vi "TH2829-20查询结果.vi"(7 "显示格式":enum16{"浮点计数法", "科学计数法"}(ring), 8 "error in":errorcluster caption="错误输入（无错误）", 9 "数量级":T1) -> (0 "error out":errorcluster caption="错误输出", 2 "judge":u8[][][](array[numeric]), 3 "result":string[][][](array[string]))   [LabVIEW 2018]
panel:
  out "read buffer":string
  out "Serial Settings:Number of Bytes at Serial Port":u32
  in  "仪器通讯端口":refnum<visa-resource-name>
  out "LED IrCompare Result":u8[][](array[numeric])
  out "LED IrResult":sgl[][](array[numeric]) format="%#_6f"
  out "总判断":u8
  out "Bls Result":sgl[][](array[numeric]) format="%#_6f"
  out "LED VfCompare Result":u8[][](array[numeric])
  out "LED VfResult":sgl[][](array[numeric]) format="%#_6f"
  out "TURN判断组合":u8[][](array[numeric])
  out "TURN数据组合":string[][](array[string])
  out "PS Compare Result":u8[][](array[numeric])
  out "Polarity Result1":string[][](array[string])
  out "Rs Compare Result":u8[][](array[numeric])
  out "Z Compare Result":u8[][](array[numeric])
  out "Balance Compare Result":u8[][](array[numeric])
  out "LxQ Compare Result":u8[][](array[numeric])
  out "DCR Compare Result":u8[][](array[numeric])
  out "C Compare Result":u8[][](array[numeric])
  out "Lk Compare Result":u8[][](array[numeric])
  out "Lx Compare Result":u8[][](array[numeric])
  out "Turns Compare Result":u8[][](array[numeric])
  out "Polarity Result":u8[][](array[numeric])
  out "Zx Result":sgl[][](array[numeric]) format="%#_6f"
  out "ACR Result":sgl[][](array[numeric]) format="%#_6f"
  out "LxQ Result":sgl[][](array[numeric]) format="%#_6f"
  out "DCR Result":sgl[][](array[numeric]) format="%#_6f"
  out "Cx Result":sgl[][](array[numeric]) format="%#_6f"
  out "Lk Result":sgl[][](array[numeric]) format="%#_6f"
  out "Lx Result":sgl[][](array[numeric]) format="%#_6f"
  out "Turns Result":sgl[][](array[numeric]) format="%#_6f"
  out "Primary Sets":string
  out "head":string
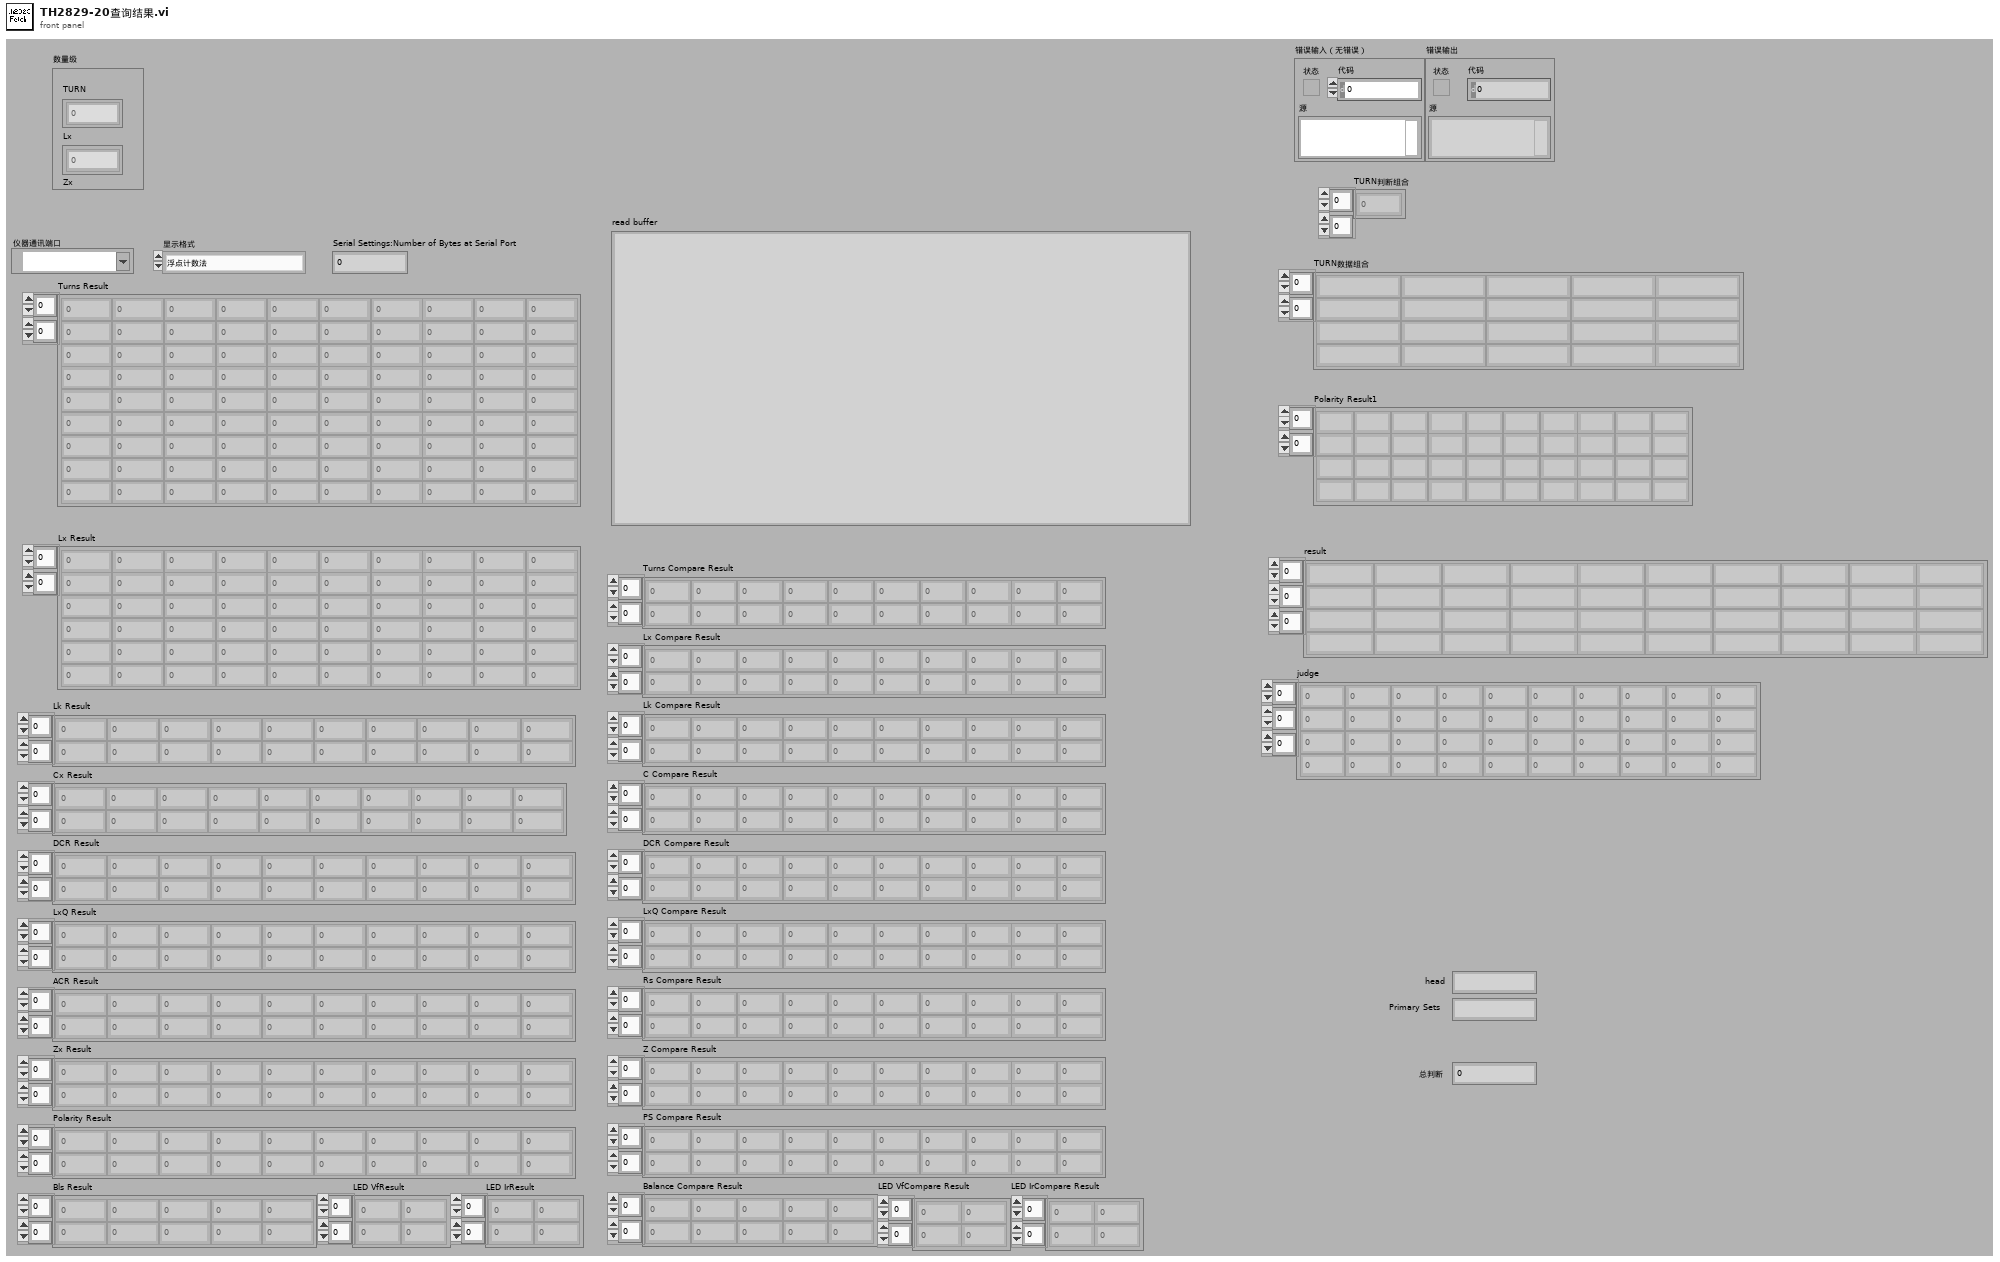
[diagram p1: front panel]
types:
  T1 = cluster{"TURN":sgl[][], "Lx":sgl[][], "Zx":sgl[][], "LK":sgl[][], "Cx":sgl[][], "ACR":sgl[][], "DCR":sgl[][], "LED+":sgl[][], "LED-":sgl[][]}
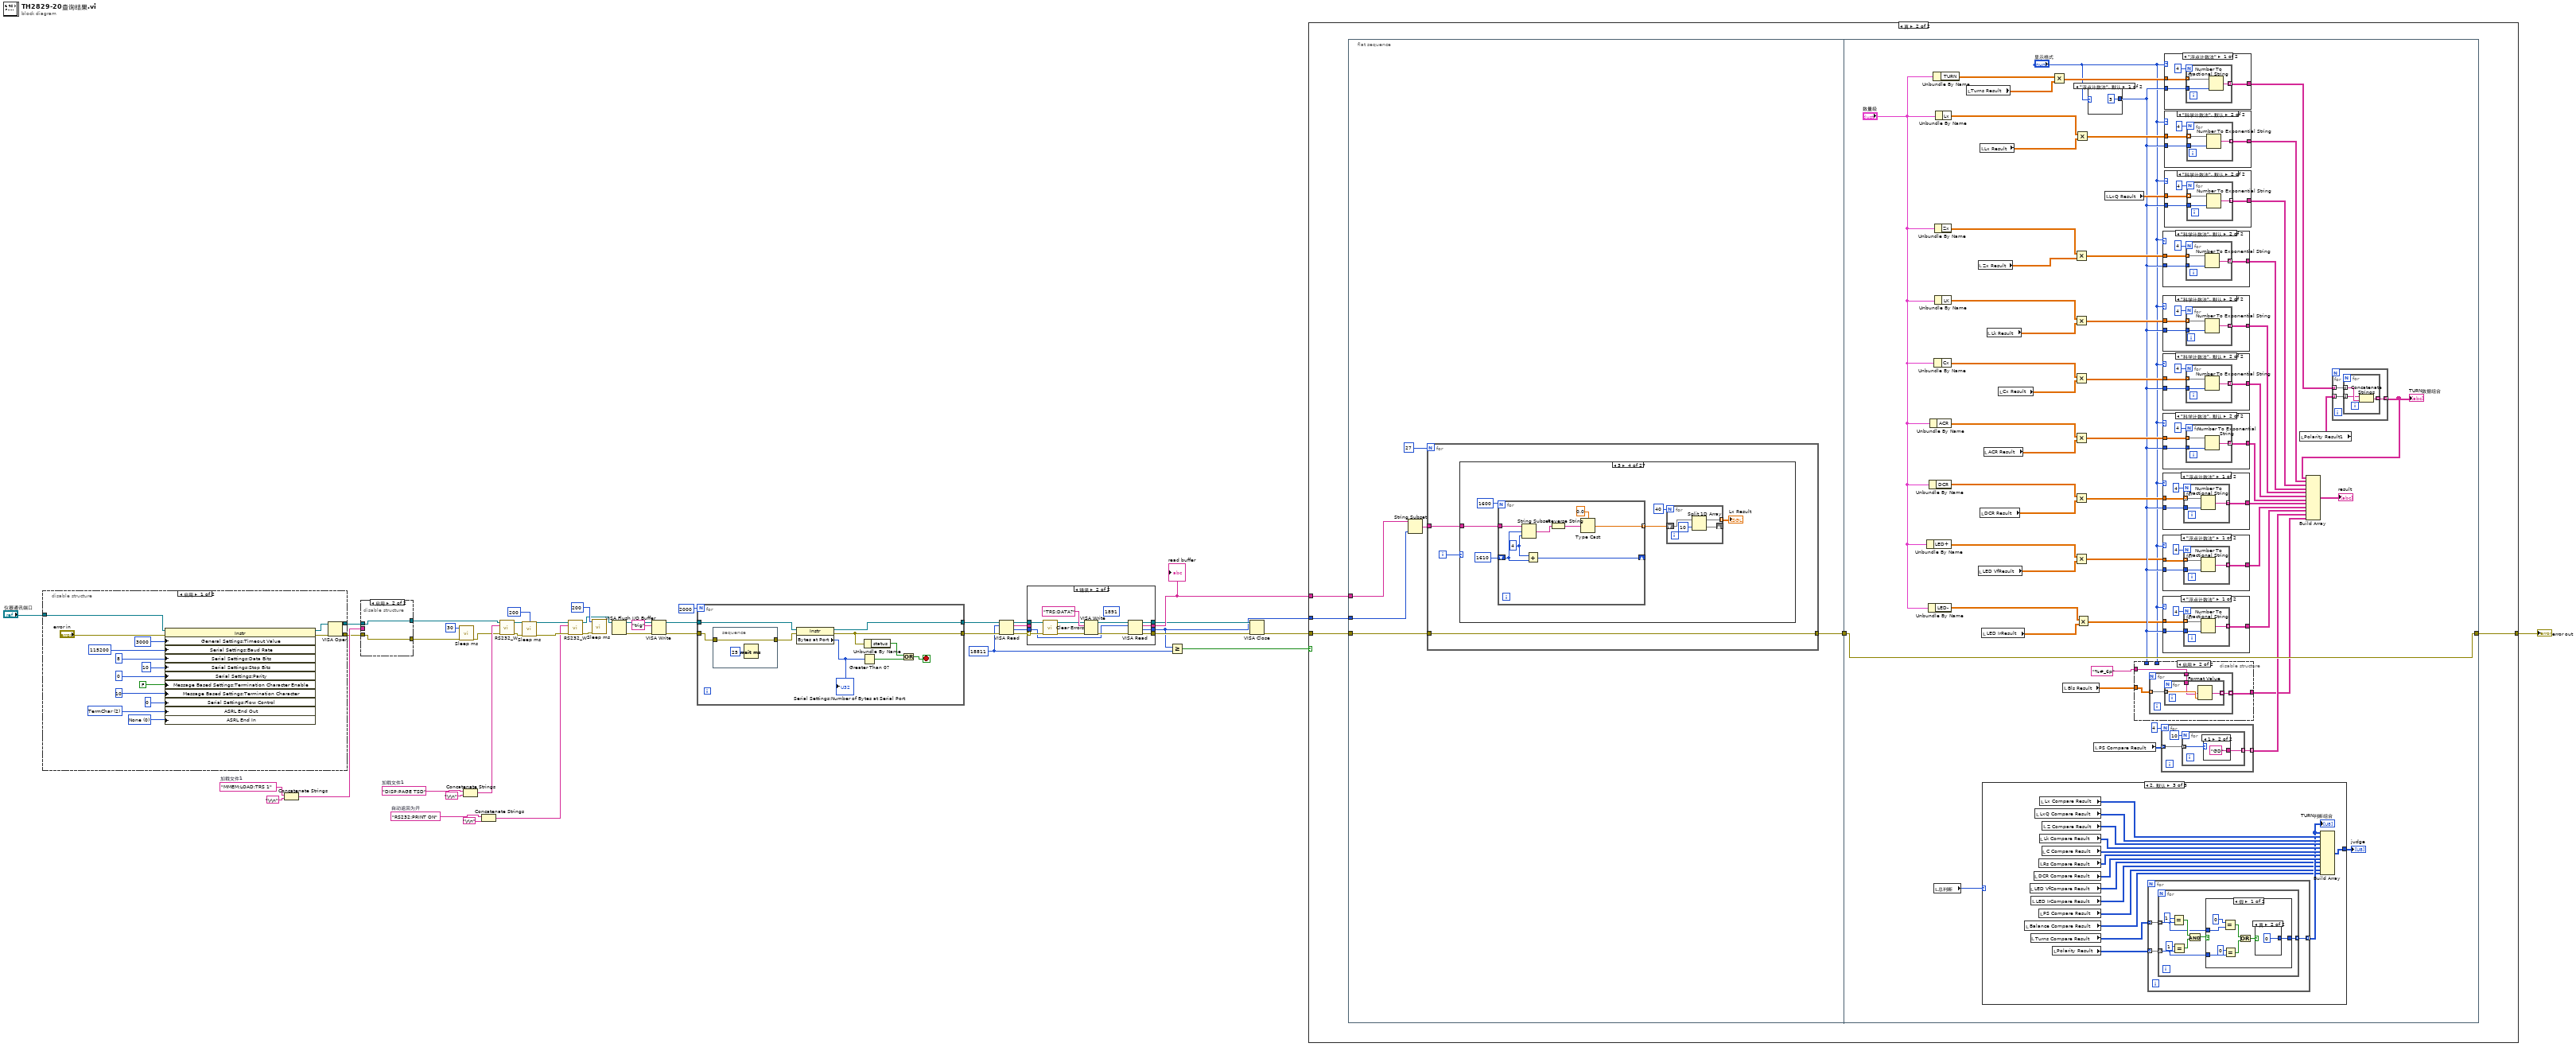
[diagram p0: block diagram]
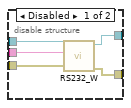
[diagram p2: hidden frame]
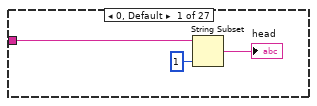
[diagram p6: hidden frame]
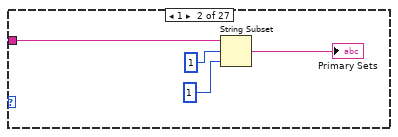
[diagram p7: hidden frame]
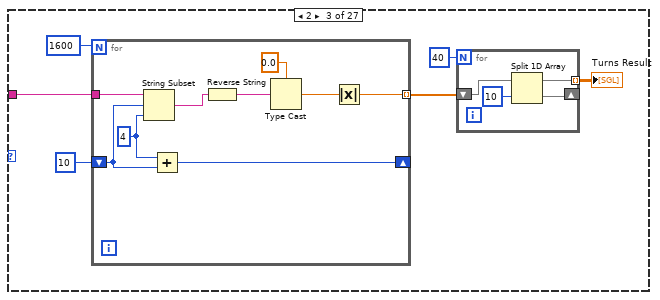
[diagram p8: hidden frame]
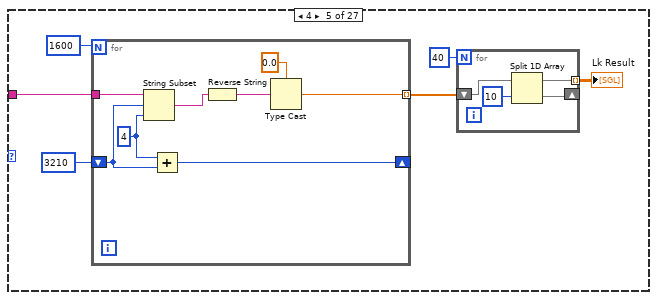
[diagram p9: hidden frame]
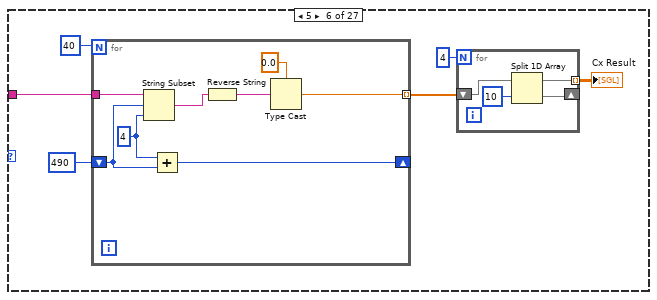
[diagram p10: hidden frame]
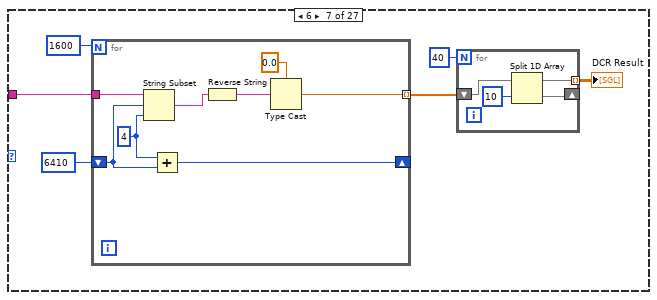
[diagram p11: hidden frame]
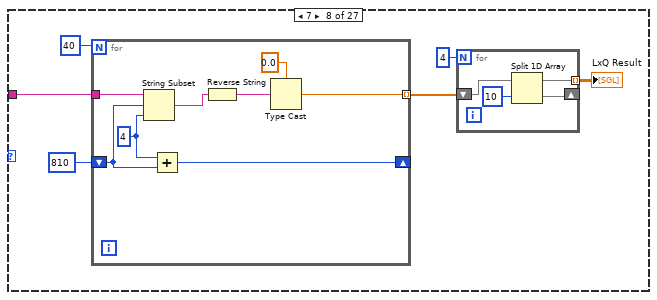
[diagram p12: hidden frame]
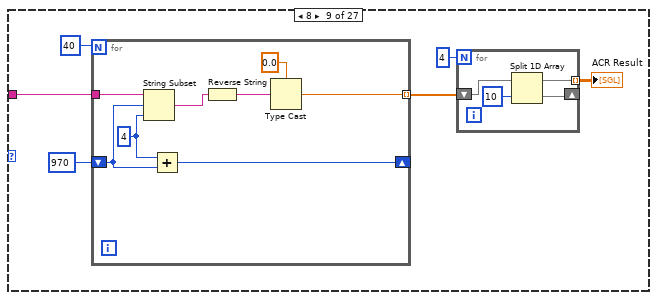
[diagram p13: hidden frame]
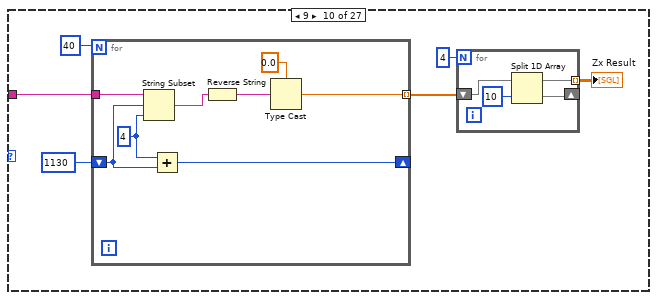
[diagram p14: hidden frame]
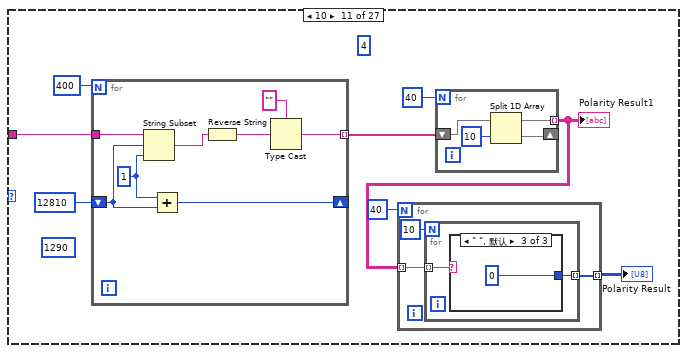
[diagram p15: hidden frame]
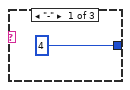
[diagram p16: hidden frame]
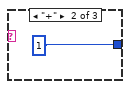
[diagram p17: hidden frame]
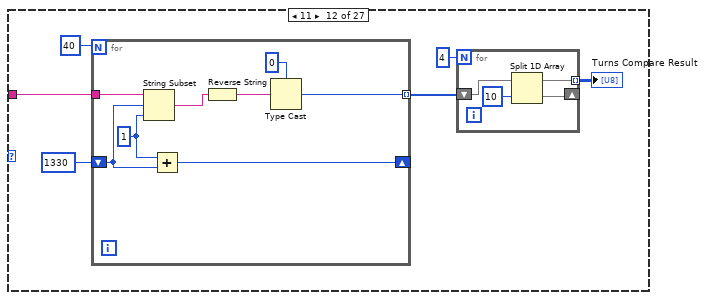
[diagram p18: hidden frame]
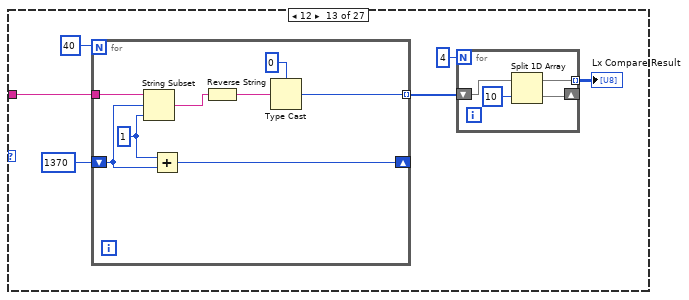
[diagram p19: hidden frame]
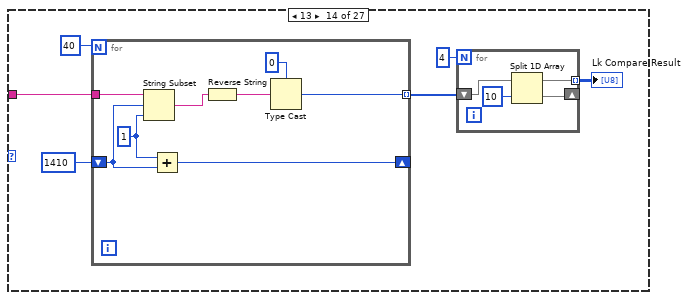
[diagram p20: hidden frame]
diagram:
  w8 = "MMEM:LOAD:TRS 1"  # 加载文件1
  w10 = "RS232:PRINT ON"  # 自动返回为开
  w11 = "DISP:PAGE TSD"  # 加载文件1
  w29 = u32 18811 ("字节总数")
  n1 = disable-structure shown="启用" {
    disable-tunnel: [w59 w60] -> w6
    disable-tunnel: [w58 _] -> w5
    disable-tunnel: "仪器通讯端口" -> [w55 w60]
    frame Enabled {
      w48 = u16 0 items=["None", "Last Bit", "TermChar"] ("Serial Settings:End Mode for Reads")
      w50 = u16 2 items=["None", "Last Bit", "TermChar", "Break"] ("Serial Settings:End Mode for Writes")
      n2 = property class="Instr"(reference=w55, error in="error in", "General Settings:Timeout Value"=u32 3000, "Serial Settings:Baud Rate"=u32 115200, "Serial Settings:Data Bits"=u16 8, "Serial Settings:Stop Bits"=u16 10, "Serial Settings:Parity"=u16 0, "Message Based Settings:Termination Character Enable"=FALSE ("TermChar En"), "Message Based Settings:Termination Character"=u8 10, "Serial Settings:Flow Control"=u16 0, "ASRL End Out"=w50, "ASRL End In"=w48) -> (reference out=w56:refnum<visa-resource-name>, error out=w57:errorcluster)
      n3 = VISA Open ("VISA打开")(error in (no error)=w57, VISA resource name=w56) -> (VISA resource name=w59:refnum<visa-resource-name>, error out=w58:errorcluster)  [unwired: 3 in]
    }
    frame Disabled {
    }
  }
  n4 = Concatenate Strings(w8, "\r\n") -> (w7:string)
  n5 = disable-structure shown="启用" {
    disable-tunnel: w7 -> [w65 _]
    disable-tunnel: w6 -> [w64 w67]
    disable-tunnel: w5 -> [w63 w66]
    disable-tunnel: [w62 w66] -> w4
    disable-tunnel: [w61 w67] -> w2
    frame Disabled {
      n6 = call "RS232_W.vi"("error in (no error)"=w63, "CMD"=w65, "VISA资源名称"=w64) -> ("error out"=w62:errorcluster, "VISA资源名称输出"=w61:refnum<visa-resource-name>)  [unwired: 6 in, 1 out]
    }
    frame Enabled {
    }
  }
  n7 = call "Sleep ms.vi"("error in (no error)"=w4, "等待时间（毫秒）"=u32 30) -> ("error out"=w1:errorcluster)  [unwired: 9 in]
  n8 = Concatenate Strings(w11, "\r\n") -> (w16:string)
  n9 = Concatenate Strings(w10, "\r\n") -> (w14:string)
  n10 = call "RS232_W.vi"("error in (no error)"=w1, "CMD"=w16, "VISA资源名称"=w2) -> ("error out"=w20:errorcluster, "VISA资源名称输出"=w17:refnum<visa-resource-name>)  [unwired: 6 in, 1 out]
  n11 = call "Sleep ms.vi"("error in (no error)"=w20, "等待时间（毫秒）"=u32 200) -> ("error out"=w21:errorcluster)  [unwired: 9 in]
  n12 = call "RS232_W.vi"("error in (no error)"=w21, "CMD"=w14, "VISA资源名称"=w17) -> ("error out"=w18:errorcluster, "VISA资源名称输出"=w13:refnum<visa-resource-name>)  [unwired: 6 in, 1 out]
  n13 = call "Sleep ms.vi"("error in (no error)"=w18, "等待时间（毫秒）"=u32 200) -> ()  [unwired: 9 in, 1 out]
  n14 = VISA Flush I/O Buffer(VISA resource name=w13) -> (VISA resource name out=w36:refnum<visa-resource-name>, error out=w37:errorcluster)  [unwired: 2 in]
  n15 = VISA Write(VISA resource name=w36, write buffer="trig", error in (no error)=w37) -> (VISA resource name out=w31:refnum<visa-resource-name>, error out=w32:errorcluster)  [unwired: 1 out]
  n16 = for {
    N: 2000 -> [_]
    tunnel: w31 -> [w76]
    tunnel: w32 -> [w68]
    tunnel: [w75] -> w34
    tunnel: [w72] -> w33
    stop <- w70 stop-if-true
    n17 = stacked-sequence {
      tunnel: [w78] -> w69
      tunnel: w68 -> [w78]
      frame #0 {
        n18 = Wait (ms)(milliseconds to wait=u32 25 ("等待时间（毫秒）")) -> ()  [unwired: 1 out]
      }
    }
    n19 = property class="Instr"(reference=w76, error in=w69) -> (reference out=w75:refnum<visa-resource-name>, error out=w72:errorcluster, "Bytes at Port"=w74:u32)
    "Serial Settings:Number of Bytes at Serial Port" <- w74
    n20 = Greater Than 0?(x=w74) -> (x > 0?=w73:bool)
    n21 = Unbundle By Name(w72) -> ("status"=w71:bool)
    n22 = Or(x=w71, y=w73) -> (x .or. y?=w70:bool)
  }
  n23 = VISA Read(VISA resource name=w34, byte count=w29, error in (no error)=w33) -> (VISA resource name out=w27:refnum<visa-resource-name>, read buffer=w25:string, return count=w26:u32, error out=w28:errorcluster)
  n24 = case shown="错误" w28 {
    selector: w28 -> [w82 w89]
    tunnel: w27 -> [w81 w88]
    tunnel: [w81 w87] -> w38
    tunnel: [w82 w86] -> w39
    tunnel: [w79 w85] -> w40
    tunnel: [w80 w84] -> w24
    tunnel: w26 -> [w80 w83]
    tunnel: w25 -> [w79 _]
    frame No Error {
    }
    frame Error {
      (unwired) u32 1891 ("字节总数")
      n25 = call <vilib>:"Clear Errors.vi"("error in (no error)"=w89) -> ("error out"=w90:errorcluster)  [unwired: 5 in, 1 out]
      n26 = VISA Write(VISA resource name=w88, write buffer="TRS:DATA?", error in (no error)=w90) -> (VISA resource name out=w92:refnum<visa-resource-name>, error out=w93:errorcluster)  [unwired: 1 out]
      n27 = VISA Read(VISA resource name=w92, byte count=w83, error in (no error)=w93) -> (VISA resource name out=w87:refnum<visa-resource-name>, read buffer=w85:string, return count=w84:u32, error out=w86:errorcluster)
    }
  }
  "read buffer" <- w40
  n28 = Greater Or Equal?(x=w24, y=w29) -> (x >= y?=w42:bool)
  n29 = VISA Close(VISA resource name=w38, error in (no error)=w39) -> (error out=w41:errorcluster)
  n30 = case shown="真" w42 {
    tunnel: w41 -> [w94 w96]
    tunnel: [w94 w99] -> w43
    tunnel: w40 -> [_ w97]
    tunnel: w24 -> [_ w95]
    frame False {
    }
    frame True {
      n31 = flat-sequence {
        tunnel: [w104] -> w98
        tunnel: w97 -> [w103]
        tunnel: w96 -> [w102]
        tunnel: w95 -> [w100]
        tunnel: [w618] -> w99
        tunnel: w98 -> [w618]
        frame #0 {
          n32 = String Subset(string=w103, length (rest)=w100) -> (substring=w105:string)  [unwired: 1 in]
          n33 = for {
            N: 27 -> [_]
            tunnel: w105 -> [w107]
            tunnel: w102 -> [w106]
            tunnel: [w106] -> w104
            i -> [w108]
            n34 = case shown="3" w108 {
              tunnel: w107 -> [w111 w115 w120 w139 w157 w175 w193 w211 w229 w247 w267 w293 w311 w329 w347 w365 w383 w401 w419 w437 w455 w472 w476 w494 w512 w530 w548]
              frame 0, Default {
                n35 = String Subset(string=w111, length (rest)=1 ("长度（剩余）")) -> (substring=→"head":string)  [unwired: 1 in]
              }
              frame 1 {
                n36 = String Subset ("截取字符串")(string=w115, offset (0)=1 ("长度（剩余）"), length (rest)=1 ("长度（剩余）")) -> (substring=→"Primary Sets":string)
              }
              frame 2 {
                n37 = for {
                  N: 1600 -> [_]
                  shift-right: [w130] -> _
                  shift-left: 10 ("长度（剩余）") -> [w126]
                  tunnel: w120 -> [w125]
                  tunnel: [w122] -> w118 mode=indexing
                  w127 = 4 ("长度（剩余）")
                  n38 = String Subset(string=w125, offset (0)=w126, length (rest)=w127) -> (substring=w124:string)
                  n39 = Add(x=w127, y=w126) -> (x+y=w130:i32)
                  n40 = Reverse String(1:w124) -> (0:w129:string)
                  n41 = Type Cast(type=sgl 0.0 ("长度（剩余）"), x=w129) -> (*(type *) &x=w123:sgl)
                  n42 = Absolute Value(x=w123) -> (abs(x)=w122:sgl)
                }
                n43 = for {
                  N: 40 -> [_]
                  shift-right: [w133] -> _
                  shift-left: w118 -> [w131]
                  tunnel: [w132] -> w116 mode=indexing
                  n44 = Split 1D Array(array=w131, index=10 ("索引")) -> (first subarray=w132:sgl[], second subarray=w133:sgl[])
                }
                "Turns Result" <- w116
              }
              frame 3 {
                n45 = for {
                  N: 1600 -> [_]
                  shift-right: [w148] -> _
                  shift-left: 1610 ("长度（剩余）") -> [w144]
                  tunnel: w139 -> [w143]
                  tunnel: [w141] -> w137 mode=indexing
                  w145 = 4 ("长度（剩余）")
                  n46 = String Subset(string=w143, offset (0)=w144, length (rest)=w145) -> (substring=w142:string)
                  n47 = Add(x=w145, y=w144) -> (x+y=w148:i32)
                  n48 = Reverse String(1:w142) -> (0:w147:string)
                  n49 = Type Cast(type=sgl 0.0 ("长度（剩余）"), x=w147) -> (*(type *) &x=w141:sgl)
                }
                n50 = for {
                  N: 40 -> [_]
                  shift-right: [w151] -> _
                  shift-left: w137 -> [w149]
                  tunnel: [w150] -> w135 mode=indexing
                  n51 = Split 1D Array(array=w149, index=10 ("索引")) -> (first subarray=w150:sgl[], second subarray=w151:sgl[])
                }
                "Lx Result" <- w135
              }
              frame 4 {
                n52 = for {
                  N: 1600 -> [_]
                  shift-right: [w166] -> _
                  shift-left: 3210 ("长度（剩余）") -> [w162]
                  tunnel: w157 -> [w161]
                  tunnel: [w159] -> w155 mode=indexing
                  w163 = 4 ("长度（剩余）")
                  n53 = String Subset(string=w161, offset (0)=w162, length (rest)=w163) -> (substring=w160:string)
                  n54 = Add(x=w163, y=w162) -> (x+y=w166:i32)
                  n55 = Reverse String(1:w160) -> (0:w165:string)
                  n56 = Type Cast(type=sgl 0.0 ("长度（剩余）"), x=w165) -> (*(type *) &x=w159:sgl)
                }
                n57 = for {
                  N: 40 -> [_]
                  shift-right: [w169] -> _
                  shift-left: w155 -> [w167]
                  tunnel: [w168] -> w153 mode=indexing
                  n58 = Split 1D Array(array=w167, index=10 ("索引")) -> (first subarray=w168:sgl[], second subarray=w169:sgl[])
                }
                "Lk Result" <- w153
              }
              frame 5 {
                n59 = for {
                  N: 40 -> [_]
                  shift-right: [w184] -> _
                  shift-left: 490 ("长度（剩余）") -> [w180]
                  tunnel: w175 -> [w179]
                  tunnel: [w177] -> w173 mode=indexing
                  w181 = 4 ("长度（剩余）")
                  n60 = String Subset(string=w179, offset (0)=w180, length (rest)=w181) -> (substring=w178:string)
                  n61 = Add(x=w181, y=w180) -> (x+y=w184:i32)
                  n62 = Reverse String(1:w178) -> (0:w183:string)
                  n63 = Type Cast(type=sgl 0.0 ("长度（剩余）"), x=w183) -> (*(type *) &x=w177:sgl)
                }
                n64 = for {
                  N: 4 -> [_]
                  shift-right: [w187] -> _
                  shift-left: w173 -> [w185]
                  tunnel: [w186] -> w171 mode=indexing
                  n65 = Split 1D Array(array=w185, index=10 ("索引")) -> (first subarray=w186:sgl[], second subarray=w187:sgl[])
                }
                "Cx Result" <- w171
              }
              frame 6 {
                n66 = for {
                  N: 1600 -> [_]
                  shift-right: [w202] -> _
                  shift-left: 6410 ("长度（剩余）") -> [w198]
                  tunnel: w193 -> [w197]
                  tunnel: [w195] -> w191 mode=indexing
                  w199 = 4 ("长度（剩余）")
                  n67 = String Subset(string=w197, offset (0)=w198, length (rest)=w199) -> (substring=w196:string)
                  n68 = Add(x=w199, y=w198) -> (x+y=w202:i32)
                  n69 = Reverse String(1:w196) -> (0:w201:string)
                  n70 = Type Cast(type=sgl 0.0 ("长度（剩余）"), x=w201) -> (*(type *) &x=w195:sgl)
                }
                n71 = for {
                  N: 40 -> [_]
                  shift-right: [w205] -> _
                  shift-left: w191 -> [w203]
                  tunnel: [w204] -> w189 mode=indexing
                  n72 = Split 1D Array(array=w203, index=10 ("索引")) -> (first subarray=w204:sgl[], second subarray=w205:sgl[])
                }
                "DCR Result" <- w189
              }
              frame 7 {
                n73 = for {
                  N: 40 -> [_]
                  shift-right: [w220] -> _
                  shift-left: 810 ("长度（剩余）") -> [w216]
                  tunnel: w211 -> [w215]
                  tunnel: [w213] -> w209 mode=indexing
                  w217 = 4 ("长度（剩余）")
                  n74 = String Subset(string=w215, offset (0)=w216, length (rest)=w217) -> (substring=w214:string)
                  n75 = Add(x=w217, y=w216) -> (x+y=w220:i32)
                  n76 = Reverse String(1:w214) -> (0:w219:string)
                  n77 = Type Cast(type=sgl 0.0 ("长度（剩余）"), x=w219) -> (*(type *) &x=w213:sgl)
                }
                n78 = for {
                  N: 4 -> [_]
                  shift-right: [w223] -> _
                  shift-left: w209 -> [w221]
                  tunnel: [w222] -> w207 mode=indexing
                  n79 = Split 1D Array(array=w221, index=10 ("索引")) -> (first subarray=w222:sgl[], second subarray=w223:sgl[])
                }
                "LxQ Result" <- w207
              }
              frame 8 {
                n80 = for {
                  N: 40 -> [_]
                  shift-right: [w238] -> _
                  shift-left: 970 ("长度（剩余）") -> [w234]
                  tunnel: w229 -> [w233]
                  tunnel: [w231] -> w227 mode=indexing
                  w235 = 4 ("长度（剩余）")
                  n81 = String Subset(string=w233, offset (0)=w234, length (rest)=w235) -> (substring=w232:string)
                  n82 = Add(x=w235, y=w234) -> (x+y=w238:i32)
                  n83 = Reverse String(1:w232) -> (0:w237:string)
                  n84 = Type Cast(type=sgl 0.0 ("长度（剩余）"), x=w237) -> (*(type *) &x=w231:sgl)
                }
                n85 = for {
                  N: 4 -> [_]
                  shift-right: [w241] -> _
                  shift-left: w227 -> [w239]
                  tunnel: [w240] -> w225 mode=indexing
                  n86 = Split 1D Array(array=w239, index=10 ("索引")) -> (first subarray=w240:sgl[], second subarray=w241:sgl[])
                }
                "ACR Result" <- w225
              }
              frame 9 {
                n87 = for {
                  N: 40 -> [_]
                  shift-right: [w256] -> _
                  shift-left: 1130 ("长度（剩余）") -> [w252]
                  tunnel: w247 -> [w251]
                  tunnel: [w249] -> w245 mode=indexing
                  w253 = 4 ("长度（剩余）")
                  n88 = String Subset(string=w251, offset (0)=w252, length (rest)=w253) -> (substring=w250:string)
                  n89 = Add(x=w253, y=w252) -> (x+y=w256:i32)
                  n90 = Reverse String(1:w250) -> (0:w255:string)
                  n91 = Type Cast(type=sgl 0.0 ("长度（剩余）"), x=w255) -> (*(type *) &x=w249:sgl)
                }
                n92 = for {
                  N: 4 -> [_]
                  shift-right: [w259] -> _
                  shift-left: w245 -> [w257]
                  tunnel: [w258] -> w243 mode=indexing
                  n93 = Split 1D Array(array=w257, index=10 ("索引")) -> (first subarray=w258:sgl[], second subarray=w259:sgl[])
                }
                "Zx Result" <- w243
              }
              frame 10 {
                (unwired) 1290 ("长度（剩余）")
                (unwired) 4
                n94 = for {
                  N: 400 -> [_]
                  shift-right: [w284] -> _
                  shift-left: 12810 ("长度（剩余）") -> [w281]
                  tunnel: w267 -> [w280]
                  tunnel: [w278] -> w262 mode=indexing
                  w282 = 1 ("长度（剩余）")
                  n95 = String Subset(string=w280, offset (0)=w281, length (rest)=w282) -> (substring=w279:string)
                  n96 = Add(x=w282, y=w281) -> (x+y=w284:i32)
                  n97 = Reverse String(1:w279) -> (0:w283:string)
                  n98 = Type Cast(type="", x=w283) -> (*(type *) &x=w278:string)
                }
                n99 = for {
                  N: 40 -> [_]
                  shift-right: [w287] -> _
                  shift-left: w262 -> [w285]
                  tunnel: [w286] -> w261 mode=indexing
                  n100 = Split 1D Array(array=w285, index=10 ("索引")) -> (first subarray=w286:string[], second subarray=w287:string[])
                }
                "Polarity Result1" <- w261
                n101 = for {
                  N: 40 -> [_]
                  tunnel: w261 -> [w270] mode=indexing
                  tunnel: [w269] -> w263 mode=indexing
                  n102 = for {
                    N: 10 -> [_]
                    tunnel: w270 -> [w273] mode=indexing
                    tunnel: [w272] -> w269 mode=indexing
                    n103 = case shown="\" \", 默认" w273 {
                      tunnel: [u8 4 u8 1 u8 0] -> w272
                      frame "-" {
                      }
                      frame "+" {
                      }
                      frame " ", Default {
                      }
                    }
                  }
                }
                "Polarity Result" <- w263
              }
              frame 11 {
                n104 = for {
                  N: 40 -> [_]
                  shift-right: [w302] -> _
                  shift-left: 1330 ("长度（剩余）") -> [w298]
                  tunnel: w293 -> [w297]
                  tunnel: [w295] -> w291 mode=indexing
                  w299 = 1 ("长度（剩余）")
                  n105 = String Subset ("截取字符串")(string=w297, offset (0)=w298, length (rest)=w299) -> (substring=w296:string)
                  n106 = Add(x=w299, y=w298) -> (x+y=w302:i32)
                  n107 = Reverse String(1:w296) -> (0:w301:string)
                  n108 = Type Cast(type=u8 0 ("长度（剩余）"), x=w301) -> (*(type *) &x=w295:u8)
                }
                n109 = for {
                  N: 4 -> [_]
                  shift-right: [w305] -> _
                  shift-left: w291 -> [w303]
                  tunnel: [w304] -> w289 mode=indexing
                  n110 = Split 1D Array(array=w303, index=10 ("索引")) -> (first subarray=w304:u8[], second subarray=w305:u8[])
                }
                "Turns Compare Result" <- w289
              }
              frame 12 {
                n111 = for {
                  N: 40 -> [_]
                  shift-right: [w320] -> _
                  shift-left: 1370 ("长度（剩余）") -> [w316]
                  tunnel: w311 -> [w315]
                  tunnel: [w313] -> w309 mode=indexing
                  w317 = 1 ("长度（剩余）")
                  n112 = String Subset(string=w315, offset (0)=w316, length (rest)=w317) -> (substring=w314:string)
                  n113 = Add(x=w317, y=w316) -> (x+y=w320:i32)
                  n114 = Reverse String(1:w314) -> (0:w319:string)
                  n115 = Type Cast(type=u8 0 ("长度（剩余）"), x=w319) -> (*(type *) &x=w313:u8)
                }
                n116 = for {
                  N: 4 -> [_]
                  shift-right: [w323] -> _
                  shift-left: w309 -> [w321]
                  tunnel: [w322] -> w307 mode=indexing
                  n117 = Split 1D Array(array=w321, index=10 ("索引")) -> (first subarray=w322:u8[], second subarray=w323:u8[])
                }
                "Lx Compare Result" <- w307
              }
              frame 13 {
                n118 = for {
                  N: 40 -> [_]
                  shift-right: [w338] -> _
                  shift-left: 1410 ("长度（剩余）") -> [w334]
                  tunnel: w329 -> [w333]
                  tunnel: [w331] -> w327 mode=indexing
                  w335 = 1 ("长度（剩余）")
                  n119 = String Subset(string=w333, offset (0)=w334, length (rest)=w335) -> (substring=w332:string)
                  n120 = Add(x=w335, y=w334) -> (x+y=w338:i32)
                  n121 = Reverse String(1:w332) -> (0:w337:string)
                  n122 = Type Cast(type=u8 0 ("长度（剩余）"), x=w337) -> (*(type *) &x=w331:u8)
                }
                n123 = for {
                  N: 4 -> [_]
                  shift-right: [w341] -> _
                  shift-left: w327 -> [w339]
                  tunnel: [w340] -> w325 mode=indexing
                  n124 = Split 1D Array(array=w339, index=10 ("索引")) -> (first subarray=w340:u8[], second subarray=w341:u8[])
                }
                "Lk Compare Result" <- w325
              }
              frame 14 {
                n125 = for {
                  N: 40 -> [_]
                  shift-right: [w356] -> _
                  shift-left: 1450 ("长度（剩余）") -> [w352]
                  tunnel: w347 -> [w351]
                  tunnel: [w349] -> w345 mode=indexing
                  w353 = 1 ("长度（剩余）")
                  n126 = String Subset(string=w351, offset (0)=w352, length (rest)=w353) -> (substring=w350:string)
                  n127 = Add(x=w353, y=w352) -> (x+y=w356:i32)
                  n128 = Reverse String(1:w350) -> (0:w355:string)
                  n129 = Type Cast(type=u8 0 ("长度（剩余）"), x=w355) -> (*(type *) &x=w349:u8)
                }
                n130 = for {
                  N: 4 -> [_]
                  shift-right: [w359] -> _
                  shift-left: w345 -> [w357]
                  tunnel: [w358] -> w343 mode=indexing
                  n131 = Split 1D Array(array=w357, index=10 ("索引")) -> (first subarray=w358:u8[], second subarray=w359:u8[])
                }
                "C Compare Result" <- w343
              }
              frame 15 {
                n132 = for {
                  N: 40 -> [_]
                  shift-right: [w374] -> _
                  shift-left: 1490 ("长度（剩余）") -> [w370]
                  tunnel: w365 -> [w369]
                  tunnel: [w367] -> w363 mode=indexing
                  w371 = 1 ("长度（剩余）")
                  n133 = String Subset(string=w369, offset (0)=w370, length (rest)=w371) -> (substring=w368:string)
                  n134 = Add(x=w371, y=w370) -> (x+y=w374:i32)
                  n135 = Reverse String(1:w368) -> (0:w373:string)
                  n136 = Type Cast(type=u8 0 ("长度（剩余）"), x=w373) -> (*(type *) &x=w367:u8)
                }
                n137 = for {
                  N: 4 -> [_]
                  shift-right: [w377] -> _
                  shift-left: w363 -> [w375]
                  tunnel: [w376] -> w361 mode=indexing
                  n138 = Split 1D Array(array=w375, index=10 ("索引")) -> (first subarray=w376:u8[], second subarray=w377:u8[])
                }
                "DCR Compare Result" <- w361
              }
              frame 16 {
                n139 = for {
                  N: 40 -> [_]
                  shift-right: [w392] -> _
                  shift-left: 1530 ("长度（剩余）") -> [w388]
                  tunnel: w383 -> [w387]
                  tunnel: [w385] -> w381 mode=indexing
                  w389 = 1 ("长度（剩余）")
                  n140 = String Subset(string=w387, offset (0)=w388, length (rest)=w389) -> (substring=w386:string)
                  n141 = Add(x=w389, y=w388) -> (x+y=w392:i32)
                  n142 = Reverse String(1:w386) -> (0:w391:string)
                  n143 = Type Cast(type=u8 0 ("长度（剩余）"), x=w391) -> (*(type *) &x=w385:u8)
                }
                n144 = for {
                  N: 4 -> [_]
                  shift-right: [w395] -> _
                  shift-left: w381 -> [w393]
                  tunnel: [w394] -> w379 mode=indexing
                  n145 = Split 1D Array(array=w393, index=10 ("索引")) -> (first subarray=w394:u8[], second subarray=w395:u8[])
                }
                "LxQ Compare Result" <- w379
              }
              frame 17 {
                n146 = for {
                  N: 40 -> [_]
                  shift-right: [w410] -> _
                  shift-left: 1570 ("长度（剩余）") -> [w404]
                  tunnel: w401 -> [w405]
                  tunnel: [w406] -> w399 mode=indexing
                  w403 = 1 ("长度（剩余）")
                  n147 = String Subset(string=w405, offset (0)=w404, length (rest)=w403) -> (substring=w407:string)
                  n148 = Add(x=w403, y=w404) -> (x+y=w410:i32)
                  n149 = Reverse String(1:w407) -> (0:w409:string)
                  n150 = Type Cast(type=u8 0 ("长度（剩余）"), x=w409) -> (*(type *) &x=w406:u8)
                }
                n151 = for {
                  N: 4 -> [_]
                  shift-right: [w413] -> _
                  shift-left: w399 -> [w411]
                  tunnel: [w412] -> w397 mode=indexing
                  n152 = Split 1D Array(array=w411, index=10 ("索引")) -> (first subarray=w412:u8[], second subarray=w413:u8[])
                }
                "Rs Compare Result" <- w397
              }
              frame 18 {
                n153 = for {
                  N: 40 -> [_]
                  shift-right: [w428] -> _
                  shift-left: 1610 ("长度（剩余）") -> [w422]
                  tunnel: w419 -> [w423]
                  tunnel: [w424] -> w417 mode=indexing
                  w421 = 1 ("长度（剩余）")
                  n154 = Add(x=w421, y=w422) -> (x+y=w428:i32)
                  n155 = String Subset(string=w423, offset (0)=w422, length (rest)=w421) -> (substring=w425:string)
                  n156 = Reverse String(1:w425) -> (0:w427:string)
                  n157 = Type Cast(type=u8 0 ("长度（剩余）"), x=w427) -> (*(type *) &x=w424:u8)
                }
                n158 = for {
                  N: 4 -> [_]
                  shift-right: [w431] -> _
                  shift-left: w417 -> [w429]
                  tunnel: [w430] -> w415 mode=indexing
                  n159 = Split 1D Array(array=w429, index=10 ("索引")) -> (first subarray=w430:u8[], second subarray=w431:u8[])
                }
                "Z Compare Result" <- w415
              }
              frame 19 {
                n160 = for {
                  N: 40 -> [_]
                  shift-right: [w446] -> _
                  shift-left: 1650 ("长度（剩余）") -> [w441]
                  tunnel: w437 -> [w442]
                  tunnel: [w443] -> w435 mode=indexing
                  w440 = 1 ("长度（剩余）")
                  n161 = String Subset(string=w442, offset (0)=w441, length (rest)=w440) -> (substring=w444:string)
                  n162 = Add(x=w440, y=w441) -> (x+y=w446:i32)
                  n163 = Reverse String(1:w444) -> (0:w445:string)
                  n164 = Type Cast(type=u8 0 ("长度（剩余）"), x=w445) -> (*(type *) &x=w443:u8)
                }
                n165 = for {
                  N: 4 -> [_]
                  shift-right: [w449] -> _
                  shift-left: w435 -> [w447]
                  tunnel: [w448] -> w433 mode=indexing
                  n166 = Split 1D Array(array=w447, index=10 ("索引")) -> (first subarray=w448:u8[], second subarray=w449:u8[])
                }
                "Balance Compare Result" <- w433
              }
              frame 20 {
                n167 = for {
                  N: 40 -> [_]
                  shift-right: [w464] -> _
                  shift-left: 1690 ("长度（剩余）") -> [w459]
                  tunnel: w455 -> [w460]
                  tunnel: [w461] -> w453 mode=indexing
                  w458 = 1 ("长度（剩余）")
                  n168 = String Subset(string=w460, offset (0)=w459, length (rest)=w458) -> (substring=w462:string)
                  n169 = Add(x=w458, y=w459) -> (x+y=w464:i32)
                  n170 = Reverse String(1:w462) -> (0:w463:string)
                  n171 = Type Cast(type=u8 0 ("长度（剩余）"), x=w463) -> (*(type *) &x=w461:u8)
                }
                n172 = for {
                  N: 4 -> [_]
                  shift-right: [w467] -> _
                  shift-left: w453 -> [w465]
                  tunnel: [w466] -> w451 mode=indexing
                  n173 = Split 1D Array(array=w465, index=10 ("索引")) -> (first subarray=w466:u8[], second subarray=w467:u8[])
                }
                "PS Compare Result" <- w451
              }
              frame 21 {
                n174 = String Subset(string=w472, offset (0)=1730 ("长度（剩余）"), length (rest)=1 ("长度（剩余）")) -> (substring=w475:string)
                n175 = Reverse String(1:w475) -> (0:w473:string)
                n176 = Type Cast(type=u8 0 ("长度（剩余）"), x=w473) -> (*(type *) &x=→"总判断":u8)
              }
              frame 22 {
                n177 = for {
                  N: 20 -> [_]
                  shift-right: [w489] -> _
                  shift-left: 1731 ("长度（剩余）") -> [w485]
                  tunnel: w476 -> [w484]
                  tunnel: [w482] -> w479 mode=indexing
                  w486 = 4 ("长度（剩余）")
                  n178 = String Subset(string=w484, offset (0)=w485, length (rest)=w486) -> (substring=w483:string)
                  n179 = Add(x=w486, y=w485) -> (x+y=w489:i32)
                  n180 = Reverse String(1:w483) -> (0:w488:string)
                  n181 = Type Cast(type=sgl 0.0 ("长度（剩余）"), x=w488) -> (*(type *) &x=w482:sgl)
                }
                n182 = for {
                  N: 4 -> [_]
                  shift-right: [w492] -> _
                  shift-left: w479 -> [w490]
                  tunnel: [w491] -> w477 mode=indexing
                  n183 = Split 1D Array(array=w490, index=5 ("索引")) -> (first subarray=w491:sgl[], second subarray=w492:sgl[])
                }
                "Bls Result" <- w477
              }
              frame 23 {
                n184 = for {
                  N: 8 -> [_]
                  shift-right: [w507] -> _
                  shift-left: 1811 ("长度（剩余）") -> [w503]
                  tunnel: w494 -> [w502]
                  tunnel: [w500] -> w496 mode=indexing
                  w504 = 4 ("长度（剩余）")
                  n185 = String Subset(string=w502, offset (0)=w503, length (rest)=w504) -> (substring=w501:string)
                  n186 = Add(x=w504, y=w503) -> (x+y=w507:i32)
                  n187 = Reverse String(1:w501) -> (0:w506:string)
                  n188 = Type Cast(type=sgl 0.0 ("长度（剩余）"), x=w506) -> (*(type *) &x=w500:sgl)
                }
                n189 = for {
                  N: 4 -> [_]
                  shift-right: [w510] -> _
                  shift-left: w496 -> [w508]
                  tunnel: [w509] -> w499 mode=indexing
                  n190 = Split 1D Array(array=w508, index=2 ("索引")) -> (first subarray=w509:sgl[], second subarray=w510:sgl[])
                }
                "LED VfResult" <- w499
              }
              frame 24 {
                n191 = for {
                  N: 8 -> [_]
                  shift-right: [w525] -> _
                  shift-left: 1843 ("长度（剩余）") -> [w521]
                  tunnel: w512 -> [w520]
                  tunnel: [w518] -> w514 mode=indexing
                  w522 = 4 ("长度（剩余）")
                  n192 = String Subset(string=w520, offset (0)=w521, length (rest)=w522) -> (substring=w519:string)
                  n193 = Add(x=w522, y=w521) -> (x+y=w525:i32)
                  n194 = Reverse String(1:w519) -> (0:w524:string)
                  n195 = Type Cast(type=sgl 0.0 ("长度（剩余）"), x=w524) -> (*(type *) &x=w518:sgl)
                }
                n196 = for {
                  N: 4 -> [_]
                  shift-right: [w528] -> _
                  shift-left: w514 -> [w526]
                  tunnel: [w527] -> w517 mode=indexing
                  n197 = Split 1D Array(array=w526, index=2 ("索引")) -> (first subarray=w527:sgl[], second subarray=w528:sgl[])
                }
                "LED IrResult" <- w517
              }
              frame 25 {
                n198 = for {
                  N: 8 -> [_]
                  shift-right: [w543] -> _
                  shift-left: 1875 ("长度（剩余）") -> [w538]
                  tunnel: w530 -> [w539]
                  tunnel: [w540] -> w532 mode=indexing
                  w537 = 1 ("长度（剩余）")
                  n199 = String Subset(string=w539, offset (0)=w538, length (rest)=w537) -> (substring=w541:string)
                  n200 = Add(x=w537, y=w538) -> (x+y=w543:i32)
                  n201 = Reverse String(1:w541) -> (0:w542:string)
                  n202 = Type Cast(type=u8 0 ("长度（剩余）"), x=w542) -> (*(type *) &x=w540:u8)
                }
                n203 = for {
                  N: 4 -> [_]
                  shift-right: [w546] -> _
                  shift-left: w532 -> [w544]
                  tunnel: [w545] -> w535 mode=indexing
                  n204 = Split 1D Array(array=w544, index=2 ("索引")) -> (first subarray=w545:u8[], second subarray=w546:u8[])
                }
                "LED VfCompare Result" <- w535
              }
              frame 26 {
                n205 = for {
                  N: 8 -> [_]
                  shift-right: [w561] -> _
                  shift-left: 1883 ("长度（剩余）") -> [w556]
                  tunnel: w548 -> [w557]
                  tunnel: [w558] -> w550 mode=indexing
                  w555 = 1 ("长度（剩余）")
                  n206 = String Subset(string=w557, offset (0)=w556, length (rest)=w555) -> (substring=w559:string)
                  n207 = Add(x=w555, y=w556) -> (x+y=w561:i32)
                  n208 = Reverse String(1:w559) -> (0:w560:string)
                  n209 = Type Cast(type=u8 0 ("长度（剩余）"), x=w560) -> (*(type *) &x=w558:u8)
                }
                n210 = for {
                  N: 4 -> [_]
                  shift-right: [w564] -> _
                  shift-left: w550 -> [w562]
                  tunnel: [w563] -> w553 mode=indexing
                  n211 = Split 1D Array(array=w562, index=2 ("索引")) -> (first subarray=w563:u8[], second subarray=w564:u8[])
                }
                "LED IrCompare Result" <- w553
              }
            }
          }
        }
        frame #1 {
          n212 = Unbundle By Name("数量级") -> ("LED+"=w574:sgl[][])
          n213 = Unbundle By Name("数量级") -> ("LED-"=w575:sgl[][])
          n214 = Unbundle By Name("数量级") -> ("DCR"=w573:sgl[][])
          n215 = Unbundle By Name("数量级") -> ("ACR"=w572:sgl[][])
          n216 = Unbundle By Name("数量级") -> ("TURN"=w578:sgl[][])
          n217 = local read "总判断"() -> (w590:u8)
          n218 = Unbundle By Name("数量级") -> ("Cx"=w571:sgl[][])
          n219 = Unbundle By Name("数量级") -> ("Zx"=w569:sgl[][])
          n220 = Unbundle By Name("数量级") -> ("LK"=w570:sgl[][])
          n221 = Unbundle By Name("数量级") -> ("Lx"=w568:sgl[][])
          n222 = local read "Turns Result"() -> (w577:sgl[][])
          n223 = local read "Zx Result"() -> (w600:sgl[][])
          n224 = local read "LED VfResult"() -> (w583:sgl[][])
          n225 = local read "Lx Result"() -> (w602:sgl[][])
          n226 = local read "DCR Result"() -> (w592:sgl[][])
          n227 = local read "LED IrResult"() -> (w580:sgl[][])
          n228 = case shown="2, 默认" w590 {
            tunnel: [w676 w681 w693] -> w609
            frame 0 {
              n229 = Initialize Array(u8 0, 10 ("维数大小"), 4 ("维数大小"), 10 ("维数大小")) -> (w676:u8[][][])
            }
            frame 1 {
              n230 = Initialize Array(u8 1, 10 ("维数大小"), 4 ("维数大小"), 10 ("维数大小")) -> (w681:u8[][][])
            }
            frame 2, Default {
              n231 = local read "Balance Compare Result"() -> (w686:u8[][])
              n232 = local read "LED VfCompare Result"() -> (w689:u8[][])
              n233 = local read "Turns Compare Result"() -> (w692:u8[][])
              n234 = local read "LED IrCompare Result"() -> (w688:u8[][])
              n235 = local read "DCR Compare Result"() -> (w694:u8[][])
              n236 = local read "LxQ Compare Result"() -> (w699:u8[][])
              n237 = local read "Rs Compare Result"() -> (w695:u8[][])
              n238 = local read "PS Compare Result"() -> (w687:u8[][])
              n239 = local read "Lk Compare Result"() -> (w697:u8[][])
              n240 = local read "Lx Compare Result"() -> (w700:u8[][])
              n241 = local read "C Compare Result"() -> (w696:u8[][])
              n242 = local read "Z Compare Result"() -> (w698:u8[][])
              n243 = local read "Polarity Result"() -> (w691:u8[][])
              n244 = for {
                tunnel: w692 -> [w703] mode=indexing
                tunnel: w691 -> [w702] mode=indexing
                tunnel: [w701] -> w690 mode=indexing
                n245 = for {
                  tunnel: w703 -> [w705] mode=indexing
                  tunnel: w702 -> [w704] mode=indexing
                  tunnel: [w706] -> w701 mode=indexing
                  n246 = Equal?(x=u8 1, y=w705) -> (x = y?=w708:bool)
                  n247 = Equal?(x=u8 1, y=w704) -> (x = y?=w707:bool)
                  n248 = And(x=w708, y=w707) -> (x .and. y?=w709:bool)
                  n249 = case shown="假" w709 {
                    tunnel: [w712 u8 1 ("x")] -> w706
                    tunnel: w705 -> [w715 _]
                    tunnel: w704 -> [w714 _]
                    frame False {
                      n250 = Equal?(x=u8 0, y=w715) -> (x = y?=w719:bool)
                      n251 = Equal?(x=u8 0, y=w714) -> (x = y?=w716:bool)
                      n252 = Or(x=w719, y=w716) -> (x .or. y?=w713:bool)
                      n253 = case shown="真" w713 {
                        tunnel: [u8 4 ("x") u8 0 ("x")] -> w712
                        frame False {
                        }
                        frame True {
                        }
                      }
                    }
                    frame True {
                    }
                  }
                }
              }
              "TURN判断组合" <- w690
              n254 = Build Array(w690, w700, w699, w698, w697, w696, w695, w694, w689, w688, w687, w686) -> (w693:u8[][][])
            }
          }
          "judge" <- w609
          n255 = local read "ACR Result"() -> (w594:sgl[][])
          n256 = local read "Lk Result"() -> (w598:sgl[][])
          n257 = local read "Cx Result"() -> (w596:sgl[][])
          n258 = Multiply(x=w578, y=w577) -> (x*y=w576:sgl[][])
          n259 = local read "Bls Result"() -> (w587:sgl[][])
          n260 = Multiply(x=w569, y=w600) -> (x*y=w601:sgl[][])
          n261 = Multiply(x=w570, y=w598) -> (x*y=w599:sgl[][])
          n262 = Multiply(x=w571, y=w596) -> (x*y=w597:sgl[][])
          n263 = Multiply(x=w572, y=w594) -> (x*y=w595:sgl[][])
          n264 = Multiply(x=w573, y=w592) -> (x*y=w593:sgl[][])
          n265 = Multiply(x=w574, y=w583) -> (x*y=w582:sgl[][])
          n266 = Multiply(x=w568, y=w602) -> (x*y=w603:sgl[][])
          n267 = Multiply(x=w575, y=w580) -> (x*y=w581:sgl[][])
          n268 = case shown="\"浮点计数法\", 默认" "显示格式" {
            tunnel: [i16 3 ("精度(6)") i16 6 ("精度(6)")] -> w588
            frame "浮点计数法", Default {
            }
            frame "科学计数法" {
            }
          }
          n269 = local read "PS Compare Result"() -> (w608:u8[][])
          n270 = local read "LxQ Result"() -> (w616:sgl[][])
          n271 = disable-structure shown="启用" {
            disable-tunnel: w588 -> [w622 _]
            disable-tunnel: w587 -> [w621 w639]
            disable-tunnel: [w620 w638] -> w584
            disable-tunnel: "显示格式" -> [w619 _]
            disable-tunnel: "%#_6p" -> [_ w637]
            frame Disabled {
              n272 = case shown="\"科学计数法\", 默认" w619 {
                tunnel: w621 -> [w625 w632]
                tunnel: [w624 w631] -> w620
                tunnel: w622 -> [w623 w630]
                frame "浮点计数法" {
                  n273 = for {
                    N: 4 -> [_]
                    tunnel: w625 -> [w629] mode=indexing
                    tunnel: [w628] -> w624 mode=indexing
                    tunnel: w623 -> [w627]
                    n274 = Number To Fractional String(number=w629, precision (6)=w627) -> (F-format string=w628:string[])  [unwired: 2 in]
                  }
                }
                frame "科学计数法", Default {
                  n275 = for {
                    N: 4 -> [_]
                    tunnel: w632 -> [w636] mode=indexing
                    tunnel: [w635] -> w631 mode=indexing
                    tunnel: w630 -> [w634]
                    n276 = Number To Exponential String(number=w636, precision (6)=w634) -> (E-format string=w635:string[])  [unwired: 2 in]
                  }
                }
              }
            }
            frame Enabled {
              n277 = for {
                tunnel: w639 -> [w642] mode=indexing
                tunnel: [w641] -> w638 mode=indexing
                tunnel: w637 -> [w640]
                n278 = for {
                  tunnel: w642 -> [w645] mode=indexing
                  tunnel: [w644] -> w641 mode=indexing
                  tunnel: w640 -> [w643]
                  n279 = Format Value(format string=w643, value (0)=w645) -> (output string=w644:string)  [unwired: 1 in]
                }
              }
            }
          }
          n280 = for {
            N: 4 -> [_]
            tunnel: w608 -> [w730] mode=indexing
            tunnel: [w729] -> w589 mode=indexing
            n281 = for {
              N: 10 -> [_]
              tunnel: w730 -> [w733] mode=indexing
              tunnel: [w732] -> w729 mode=indexing
              n282 = case shown="1" w733 {
                tunnel: ["NG" "GD"] -> w732
                frame 0, Default {
                }
                frame 1 {
                }
              }
            }
          }
          n283 = case shown="\"浮点计数法\"" "显示格式" {
            tunnel: w593 -> [w738 w745]
            tunnel: [w737 w744] -> w613
            tunnel: w588 -> [w736 w743]
            frame "浮点计数法" {
              n284 = for {
                N: 4 -> [_]
                tunnel: w738 -> [w742] mode=indexing
                tunnel: [w741] -> w737 mode=indexing
                tunnel: w736 -> [w740]
                n285 = Number To Fractional String(number=w742, precision (6)=w740) -> (F-format string=w741:string[])  [unwired: 2 in]
              }
            }
            frame "科学计数法", Default {
              n286 = for {
                N: 4 -> [_]
                tunnel: w745 -> [w749] mode=indexing
                tunnel: [w748] -> w744 mode=indexing
                tunnel: w743 -> [w747]
                n287 = Number To Exponential String(number=w749, precision (6)=w747) -> (E-format string=w748:string[])  [unwired: 2 in]
              }
            }
          }
          n288 = case shown="\"浮点计数法\"" "显示格式" {
            tunnel: w582 -> [w664 w671]
            tunnel: [w663 w670] -> w586
            tunnel: w588 -> [w662 w669]
            frame "浮点计数法" {
              n289 = for {
                N: 4 -> [_]
                tunnel: w664 -> [w668] mode=indexing
                tunnel: [w667] -> w663 mode=indexing
                tunnel: w662 -> [w666]
                n290 = Number To Fractional String(number=w668, precision (6)=w666) -> (F-format string=w667:string[])  [unwired: 2 in]
              }
            }
            frame "科学计数法", Default {
              n291 = for {
                N: 4 -> [_]
                tunnel: w671 -> [w675] mode=indexing
                tunnel: [w674] -> w670 mode=indexing
                tunnel: w669 -> [w673]
                n292 = Number To Exponential String(number=w675, precision (6)=w673) -> (E-format string=w674:string[])  [unwired: 2 in]
              }
            }
          }
          n293 = case shown="\"浮点计数法\"" "显示格式" {
            tunnel: w581 -> [w650 w657]
            tunnel: [w649 w656] -> w585
            tunnel: w588 -> [w648 w655]
            frame "浮点计数法" {
              n294 = for {
                N: 4 -> [_]
                tunnel: w650 -> [w654] mode=indexing
                tunnel: [w653] -> w649 mode=indexing
                tunnel: w648 -> [w652]
                n295 = Number To Fractional String(number=w654, precision (6)=w652) -> (F-format string=w653:string[])  [unwired: 2 in]
              }
            }
            frame "科学计数法", Default {
              n296 = for {
                N: 4 -> [_]
                tunnel: w657 -> [w661] mode=indexing
                tunnel: [w660] -> w656 mode=indexing
                tunnel: w655 -> [w659]
                n297 = Number To Exponential String(number=w661, precision (6)=w659) -> (E-format string=w660:string[])  [unwired: 2 in]
              }
            }
          }
          n298 = case shown="\"科学计数法\", 默认" "显示格式" {
            tunnel: w601 -> [w794 w801]
            tunnel: [w793 w800] -> w614
            tunnel: w588 -> [w792 w799]
            frame "浮点计数法" {
              n299 = for {
                N: 4 -> [_]
                tunnel: w794 -> [w798] mode=indexing
                tunnel: [w797] -> w793 mode=indexing
                tunnel: w792 -> [w796]
                n300 = Number To Fractional String(number=w798, precision (6)=w796) -> (F-format string=w797:string[])  [unwired: 2 in]
              }
            }
            frame "科学计数法", Default {
              n301 = for {
                N: 4 -> [_]
                tunnel: w801 -> [w805] mode=indexing
                tunnel: [w804] -> w800 mode=indexing
                tunnel: w799 -> [w803]
                n302 = Number To Exponential String(number=w805, precision (6)=w803) -> (E-format string=w804:string[])  [unwired: 2 in]
              }
            }
          }
          n303 = case shown="\"科学计数法\", 默认" "显示格式" {
            tunnel: w599 -> [w780 w787]
            tunnel: [w779 w786] -> w610
            tunnel: w588 -> [w778 w785]
            frame "浮点计数法" {
              n304 = for {
                N: 4 -> [_]
                tunnel: w780 -> [w784] mode=indexing
                tunnel: [w783] -> w779 mode=indexing
                tunnel: w778 -> [w782]
                n305 = Number To Fractional String(number=w784, precision (6)=w782) -> (F-format string=w783:string[])  [unwired: 2 in]
              }
            }
            frame "科学计数法", Default {
              n306 = for {
                N: 4 -> [_]
                tunnel: w787 -> [w791] mode=indexing
                tunnel: [w790] -> w786 mode=indexing
                tunnel: w785 -> [w789]
                n307 = Number To Exponential String(number=w791, precision (6)=w789) -> (E-format string=w790:string[])  [unwired: 2 in]
              }
            }
          }
          n308 = case shown="\"科学计数法\", 默认" "显示格式" {
            tunnel: w597 -> [w766 w773]
            tunnel: [w765 w772] -> w611
            tunnel: w588 -> [w764 w771]
            frame "浮点计数法" {
              n309 = for {
                N: 4 -> [_]
                tunnel: w766 -> [w770] mode=indexing
                tunnel: [w769] -> w765 mode=indexing
                tunnel: w764 -> [w768]
                n310 = Number To Fractional String(number=w770, precision (6)=w768) -> (F-format string=w769:string[])  [unwired: 2 in]
              }
            }
            frame "科学计数法", Default {
              n311 = for {
                N: 4 -> [_]
                tunnel: w773 -> [w777] mode=indexing
                tunnel: [w776] -> w772 mode=indexing
                tunnel: w771 -> [w775]
                n312 = Number To Exponential String(number=w777, precision (6)=w775) -> (E-format string=w776:string[])  [unwired: 2 in]
              }
            }
          }
          n313 = case shown="\"科学计数法\", 默认" "显示格式" {
            tunnel: w595 -> [w752 w759]
            tunnel: [w751 w758] -> w612
            tunnel: w588 -> [w750 w757]
            frame "浮点计数法" {
              n314 = for {
                N: 4 -> [_]
                tunnel: w752 -> [w756] mode=indexing
                tunnel: [w755] -> w751 mode=indexing
                tunnel: w750 -> [w754]
                n315 = Number To Fractional String(number=w756, precision (6)=w754) -> (F-format string=w755:string[])  [unwired: 2 in]
              }
            }
            frame "科学计数法", Default {
              n316 = for {
                N: 4 -> [_]
                tunnel: w759 -> [w763] mode=indexing
                tunnel: [w762] -> w758 mode=indexing
                tunnel: w757 -> [w761]
                n317 = Number To Exponential String(number=w763, precision (6)=w761) -> (E-format string=w762:string[])  [unwired: 2 in]
              }
            }
          }
          n318 = case shown="\"浮点计数法\"" "显示格式" {
            tunnel: w576 -> [w836 w843]
            tunnel: [w835 w842] -> w606
            tunnel: w588 -> [w834 w841]
            frame "浮点计数法" {
              n319 = for {
                N: 4 -> [_]
                tunnel: w836 -> [w840] mode=indexing
                tunnel: [w839] -> w835 mode=indexing
                tunnel: w834 -> [w838]
                n320 = Number To Fractional String(number=w840, precision (6)=w838) -> (F-format string=w839:string[])  [unwired: 2 in]
              }
            }
            frame "科学计数法", Default {
              n321 = for {
                N: 4 -> [_]
                tunnel: w843 -> [w847] mode=indexing
                tunnel: [w846] -> w842 mode=indexing
                tunnel: w841 -> [w845]
                n322 = Number To Exponential String(number=w847, precision (6)=w845) -> (E-format string=w846:string[])  [unwired: 2 in]
              }
            }
          }
          n323 = case shown="\"科学计数法\", 默认" "显示格式" {
            tunnel: w603 -> [w822 w829]
            tunnel: [w821 w828] -> w617
            tunnel: w588 -> [w820 w827]
            frame "浮点计数法" {
              n324 = for {
                N: 4 -> [_]
                tunnel: w822 -> [w826] mode=indexing
                tunnel: [w825] -> w821 mode=indexing
                tunnel: w820 -> [w824]
                n325 = Number To Fractional String(number=w826, precision (6)=w824) -> (F-format string=w825:string[])  [unwired: 2 in]
              }
            }
            frame "科学计数法", Default {
              n326 = for {
                N: 4 -> [_]
                tunnel: w829 -> [w833] mode=indexing
                tunnel: [w832] -> w828 mode=indexing
                tunnel: w827 -> [w831]
                n327 = Number To Exponential String(number=w833, precision (6)=w831) -> (E-format string=w832:string[])  [unwired: 2 in]
              }
            }
          }
          n328 = case shown="\"科学计数法\", 默认" "显示格式" {
            tunnel: w616 -> [w808 w815]
            tunnel: [w807 w814] -> w615
            tunnel: w588 -> [w806 w813]
            frame "浮点计数法" {
              n329 = for {
                N: 4 -> [_]
                tunnel: w808 -> [w812] mode=indexing
                tunnel: [w811] -> w807 mode=indexing
                tunnel: w806 -> [w810]
                n330 = Number To Fractional String(number=w812, precision (6)=w810) -> (F-format string=w811:string[])  [unwired: 2 in]
              }
            }
            frame "科学计数法", Default {
              n331 = for {
                N: 4 -> [_]
                tunnel: w815 -> [w819] mode=indexing
                tunnel: [w818] -> w814 mode=indexing
                tunnel: w813 -> [w817]
                n332 = Number To Exponential String(number=w819, precision (6)=w817) -> (E-format string=w818:string[])  [unwired: 2 in]
              }
            }
          }
          n333 = local read "Polarity Result1"() -> (w605:string[][])
          n334 = for {
            tunnel: w606 -> [w725] mode=indexing
            tunnel: w605 -> [w724] mode=indexing
            tunnel: [w723] -> w604 mode=indexing
            n335 = for {
              tunnel: w725 -> [w727] mode=indexing
              tunnel: w724 -> [w726] mode=indexing
              tunnel: [w728] -> w723 mode=indexing
              n336 = Concatenate Strings(w726, w727) -> (w728:string)
            }
          }
          "TURN数据组合" <- w604
          n337 = Build Array(w604, w617, w615, w614, w610, w611, w612, w613, w586, w585, w589, w584) -> (→"result":string[][][])
        }
      }
    }
  }
  "error out" <- w43
